vi "Start camera.vi"() -> ()   [LabVIEW 2012]
panel:
  out "Camera Handle":u32
  in  "Camera device ID":dbl
  out "Number of cameras":dbl
  out "error out":errorcluster
  in  "error in (no error)":errorcluster
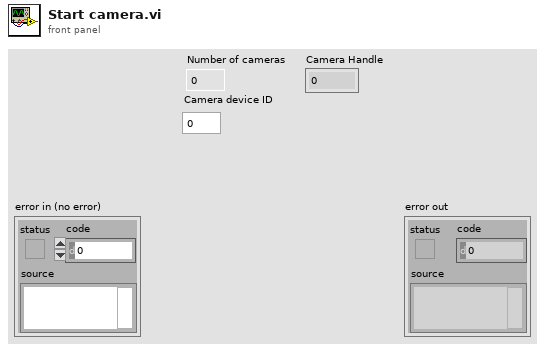
[diagram p1: front panel]
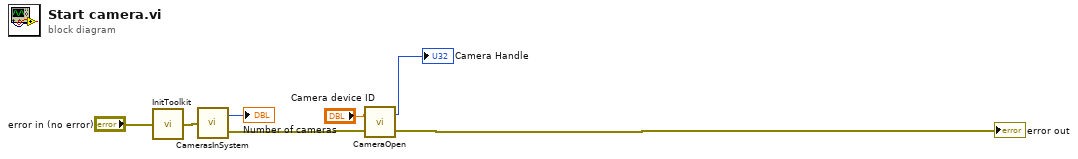
[diagram p0: block diagram]
diagram:
  n1 = call <userlib>:"InitToolkit.vi"("error in"="error in (no error)") -> ("error out"=w6:errorcluster)
  n2 = call <userlib>:"CamerasInSystem.vi"("error in"=w6) -> ("Number of Cameras"=→"Number of cameras":i32, "error out"=w4:errorcluster)
  n3 = call <userlib>:"CameraOpen.vi"("error in"=w4, "Camera Device ID"="Camera device ID") -> ("error out"=→"error out":errorcluster, "Camera Handle"=→"Camera Handle":u32)
